vi "WritePixelRgbaU64.vi"(7 "Pixel value":T1, 8 "error in":errorcluster, 9 "Y Coordinate":i32, 10 "X Coordinate":i32, 11 "Image Reference In":T2) -> (0 "error out":errorcluster, 3 "Image Reference Out":T2)   [LabVIEW 2024, in "OpenLvVision_Image.lvlib" / "DataAccess.lvlib"]
doc: "Write the pixel's value at the given coordinates."
uses:
  DataAccess.lvlib
  Management/TypeDef/Image.ctl
  <vilib>/Utility/error.llb/Error Cluster From Error Code.vi
  <vilib>/ErrorRing/Error Ring.xnode
  Management/Management.lvlib
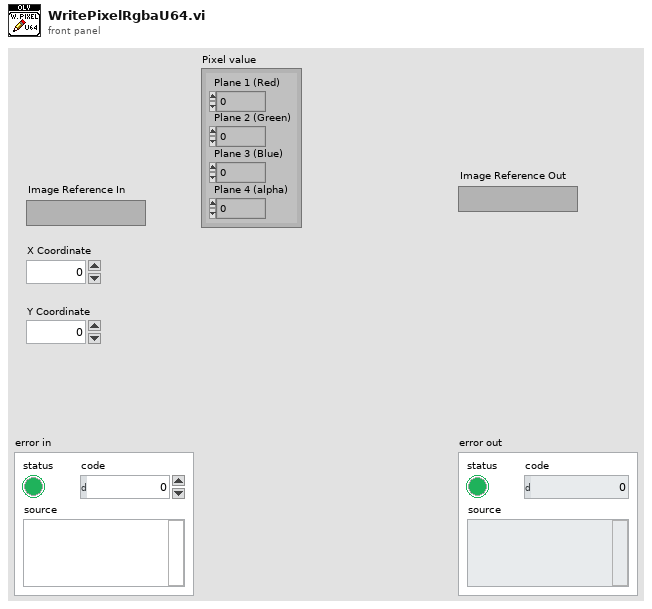
[diagram p1: front panel]
types:
  T1 = typedef "Color (U64)" = cluster{"Plane 3 (Blue)":u16, "Plane 2 (Green)":u16, "Plane 1 (Red)":u16, "Plane 4 (alpha)":u16}
  T2 = typedef "OpenLvVision_Image.lvlib/Management.lvlib/Image.ctl" = refnum<image>
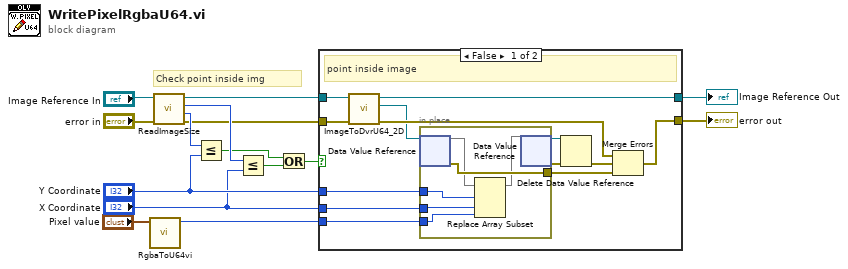
[diagram p0: block diagram]
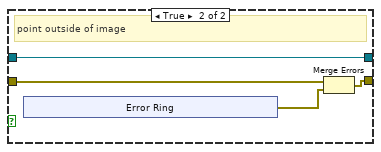
[diagram p2: hidden frame]
diagram:
  # "Check point inside img"
  n1 = call "RgbaToU64vi.vi"("Rgba"="Pixel value") -> ("U64"=w1:u64)  [unwired: 10 in]
  n2 = call "ReadImageSize.vi"("error in"="error in", "Image Reference In"="Image Reference In") -> ("error out"=w5:errorcluster, "Height"=w11:i32, "Width"=w13:i32, "Image Reference Out"=w12:T2)  [unwired: 6 in]
  n3 = Less Or Equal?(x=w11, y="Y Coordinate") -> (x <= y?=w9:bool)
  n4 = Less Or Equal?(x=w13, y="X Coordinate") -> (x <= y?=w10:bool)
  n5 = Or(x=w9, y=w10) -> (x .or. y?=w8:bool)
  n6 = case shown="False" w8 {
    tunnel: w12 -> [w28 w36]
    tunnel: w5 -> [w27 w38]
    tunnel: "Y Coordinate" -> [w19 _]
    tunnel: "X Coordinate" -> [w18 _]
    tunnel: [w26 w36] -> w4
    tunnel: [w17 w35] -> w3
    tunnel: w1 -> [w16 _]
    frame False {
      # "point inside image"
      n7 = call "ImageToDvrU64_2D.vi"("error in"=w27, "Image Reference In"=w28) -> ("error out"=w21:errorcluster, "EDVR 2D U64"=w20:refnum<data-value>, "Image Reference Out"=w26:T2)  [unwired: 6 in, 1 out]
      n8 = in-place {
        in-place-border: [w34] -> w24
        in-place-border: w19 -> [w30]
        in-place-border: w18 -> [w31]
        in-place-border: w16 -> [w29]
        n9 = in-place-dvr #1(w20) -> (w33:u64[][], w34:errorcluster)
        n10 = Replace Array Subset(array=w33, new element=w29, index (row)=w30, index (col)=w31) -> (w32:u64[][])
        n11 = in-place-dvr #1(w32) -> (w22:refnum<data-value>, w23:errorcluster)
      }
      n12 = Delete Data Value Reference(data value reference=w22, error in=w23) -> (error out=w25:errorcluster)  [unwired: 1 out]
      n13 = Merge Errors(w21, w25, w24) -> (w17:errorcluster)
    }
    frame True {
      # "point outside of image"
      n14 = xnode "Error Ring"() -> ("error out"=w37:errorcluster)
      n15 = Merge Errors(w38, w37) -> (w35:errorcluster)
    }
  }
  "error out" <- w3
  "Image Reference Out" <- w4
